vi "rsidr_core_global.vi"() -> ()   [LabVIEW 2020, in "Rohde&Schwarz RTx Oscilloscopes.lvlib"] (continued)
"Access"=0, "Range Table"="", "Read Callback"="rsrtx_FormatLINFrameRepCapInt_ReadCallback.vi", "Write Callback"="", "Supported Models"="", "Instrument Options"="", "Flags"=0, "Help"="Returns the checksum value.\n\nAvailable Repeated Capabilities:\nSerialBus: SB1, SB2, SB3, SB4\r\n\nRemote-control command(s):\nBUS<b>:LIN:FRAMe<n>:CSValue?"}, {"Level"=3, "Class Only"=FALSE, "Identifier"="RSRTX_ATTR_PROTOCOL_LIN_FRAME_PARITY_ENABLED", "Descriptive Name"="Protocol LIN Frame Parity Enabled", "Data Type"=0, "Command"="BUS{SerialBus}:LIN:FRAM<Frame>:IDST?", "Access"=0, "Range Table"="rsrtx_rngLINParity", "Read Callback"="rsrtx_FormatLINFrameRepCapInt_ReadCallback.vi", "Write Callback"="", "Supported Models"="", "Instrument Options"="", "Flags"=0, "Help"="Returns the identifier state of the selected frame.\n\nAvailable Repeated Capabilities:\nSerialBus: SB1, SB2, SB3, SB4\r\n\nRemote-control command(s):\nBUS<b>:LIN:FRAMe<n>:IDSTate?"}, {"Level"=3, "Class Only"=FALSE, "Identifier"="RSRTX_ATTR_PROTOCOL_LIN_FRAME_PARITY_VALUE", "Descriptive Name"="Protocol LIN Frame Parity Value", "Data Type"=0, "Command"="BUS{SerialBus}:LIN:FRAM<Frame>:IDPV?", "Access"=0, "Range Table"="", "Read Callback"="rsrtx_FormatLINFrameRepCapInt_ReadCallback.vi", "Write Callback"="", "Supported Models"="", "Instrument Options"="", "Flags"=0, "Help"="Returns the parity value.\n\nAvailable Repeated Capabilities:\nSerialBus: SB1, SB2, SB3, SB4\r\n\nRemote-control command(s):\nBUS<b>:LIN:FRAMe<n>:IDPValue?"}, {"Level"=3, "Class Only"=FALSE, "Identifier"="RSRTX_ATTR_PROTOCOL_LIN_FRAME_ID_VALUE", "Descriptive Name"="Protocol LIN Frame ID Value", "Data Type"=0, "Command"="BUS{SerialBus}:LIN:FRAM<Frame>:IDV?", "Access"=0, "Range Table"="", "Read Callback"="rsrtx_FormatLINFrameRepCapInt_ReadCallback.vi", "Write Callback"="", "Supported Models"="", "Instrument Options"="", "Flags"=0, "Help"="Returns the identifier value (address).\n\nAvailable Repeated Capabilities:\nSerialBus: SB1, SB2, SB3, SB4\r\n\nRemote-control command(s):\nBUS<b>:LIN:FRAMe<n>:IDValue?"}, {"Level"=3, "Class Only"=FALSE, "Identifier"="RSRTX_ATTR_PROTOCOL_LIN_FRAME_SYNC_ENABLED", "Descriptive Name"="Protocol LIN Frame Sync Enabled", "Data Type"=0, "Command"="BUS{SerialBus}:LIN:FRAM<Frame>:SYST?", "Access"=0, "Range Table"="rsrtx_rngLINChecksum", "Read Callback"="rsrtx_FormatLINFrameRepCapInt_ReadCallback.vi", "Write Callback"="", "Supported Models"="", "Instrument Options"="", "Flags"=0, "Help"="Returns the state of the sync field for the specified frame.\n\nAvailable Repeated Capabilities:\nSerialBus: SB1, SB2, SB3, SB4\r\n\nRemote-control command(s):\nBUS<b>:LIN:FRAMe<n>:SYSTate?"}, {"Level"=3, "Class Only"=FALSE, "Identifier"="RSRTX_ATTR_PROTOCOL_LIN_FRAME_SYNC_VALUE", "Descriptive Name"="Protocol LIN Frame Sync Value", "Data Type"=0, "Command"="BUS{SerialBus}:LIN:FRAM<Frame>:SYV?", "Access"=0, "Range Table"="", "Read Callback"="rsrtx_FormatLINFrameRepCapInt_ReadCallback.vi", "Write Callback"="", "Supported Models"="", "Instrument Options"="", "Flags"=0, "Help"="Returns the value of the synchronization field.\n\nAvailable Repeated Capabilities:\nSerialBus: SB1, SB2, SB3, SB4\r\n\nRemote-control command(s):\nBUS<b>:LIN:FRAMe<n>:SYValue?"}, {"Level"=3, "Class Only"=FALSE, "Identifier"="RSRTX_ATTR_PROTOCOL_LIN_FRAME_VERSION", "Descriptive Name"="Protocol LIN Frame Version", "Data Type"=0, "Command"="BUS{SerialBus}:LIN:FRAM<Frame>:VERS?", "Access"=0, "Range Table"="rsrtx_rngLINFrameVersion", "Read Callback"="rsrtx_FormatLINFrameRepCapInt_ReadCallback.vi", "Write Callback"="", "Supported Models"="", "Instrument Options"="", "Flags"=0, "Help"="Returns the version of the LIN standard for the specified frame.\n\nAvailable Repeated Capabilities:\nSerialBus: SB1, SB2, SB3, SB4\r\n\nRemote-control command(s):\nBUS<b>:LIN:FRAMe<n>:VERSion?"}, {"Level"=3, "Class Only"=FALSE, "Identifier"="RSRTX_ATTR_PROTOCOL_LIN_BYTE_COUNT", "Descriptive Name"="Protocol LIN Byte Count", "Data Type"=0, "Command"="BUS{SerialBus}:LIN:FRAM<Frame>:BCO?", "Access"=0, "Range Table"="", "Read Callback"="rsrtx_FormatLINFrameRepCapInt_ReadCallback.vi", "Write Callback"="", "Supported Models"="", "Instrument Options"="", "Flags"=0, "Help"="Returns the number of data bytes in the specified frame.\n\nAvailable Repeated Capabilities:\nSerialBus: SB1, SB2, SB3, SB4\r\n\nRemote-control command(s):\nBUS<b>:LIN:FRAMe<n>:BCOunt?"}, {"Level"=3, "Class Only"=FALSE, "Identifier"="RSRTX_ATTR_PROTOCOL_LIN_SELECTED_BYTE", "Descriptive Name"="Protocol LIN Selected Byte", "Data Type"=0, "Command"="", "Access"=2, "Range Table"="", "Read Callback"="", "Write Callback"="", "Supported Models"="", "Instrument Options"="", "Flags"=0, "Help"="Sets selector repeated capability Byte.\n\nAvailable Repeated Capabilities:\nNone\n\nRemote-control command(s):\n"}, {"Level"=3, "Class Only"=FALSE, "Identifier"="RSRTX_ATTR_PROTOCOL_LIN_BYTE_ENABLED", "Descriptive Name"="Protocol LIN Byte Enabled", "Data Type"=0, "Command"="BUS{SerialBus}:LIN:FRAM<Frame>:BYTE<Byte>:STAT?", "Access"=0, "Range Table"="rsrtx_rngLINByteEnabled", "Read Callback"="rsrtx_FormatLINFrameByteRepCapInt_ReadCallback.vi", "Write Callback"="", "Supported Models"="", "Instrument Options"="", "Flags"=0, "Help"="Returns the state of the specified data byte.\n\nAvailable Repeated Capabilities:\nSerialBus: SB1, SB2, SB3, SB4\r\n\nRemote-control command(s):\nBUS<b>:LIN:FRAMe<n>:BYTE<o>:STATe?"}, {"Level"=3, "Class Only"=FALSE, "Identifier"="RSRTX_ATTR_PROTOCOL_LIN_BYTE_VALUE", "Descriptive Name"="Protocol LIN Byte Value", "Data Type"=0, "Command"="BUS{SerialBus}:LIN:FRAM<Frame>:BYTE<Byte>:VAL?", "Access"=0, "Range Table"="", "Read Callback"="rsrtx_FormatLINFrameByteRepCapInt_ReadCallback.vi", "Write Callback"="", "Supported Models"="", "Instrument Options"="", "Flags"=0, "Help"="Returns the decimal value of the specified byte.\n\nAvailable Repeated Capabilities:\nSerialBus: SB1, SB2, SB3, SB4\r\n\nRemote-control command(s):\nBUS<b>:LIN:FRAMe<n>:BYTE<o>:VALue?"}, {"Level"=2, "Class Only"=TRUE, "Identifier"="", "Descriptive Name"="CAN", "Data Type"=0, "Command"="", "Access"=0, "Range Table"="", "Read Callback"="", "Write Callback"="", "Supported Models"="", "Instrument Options"="", "Flags"=0, "Help"="This class contains attributes that configure the CAN (Controller Area Network)\n\nAttributes in this class requires option K3."}, {"Level"=3, "Class Only"=FALSE, "Identifier"="RSRTX_ATTR_PROTOCOL_CAN_LINE_TYPE", "Descriptive Name"="Protocol CAN Line Type", "Data Type"=0, "Command"="BUS{SerialBus}:CAN:TYPE", "Access"=2, "Range Table"="rsrtx_rngProtocolCANLineType", "Read Callback"="", "Write Callback"="", "Supported Models"="", "Instrument Options"="K3", "Flags"=0, "Help"="Configures input channel of the CAN line.\n\nAvailable Repeated Capabilities:\nSerialBus: SB1, SB2, SB3, SB4\r\n\nRemote-control command(s):\nBUS<b>:CAN:TYPE"}, {"Level"=3, "Class Only"=FALSE, "Identifier"="RSRTX_ATTR_PROTOCOL_CAN_SOURCE", "Descriptive Name"="Protocol CAN Source", "Data Type"=0, "Command"="BUS{SerialBus}:CAN:DATA:SOUR", "Access"=2, "Range Table"="RsRtx_rngChannelAndDigitalSource", "Read Callback"="", "Write Callback"="", "Supported Models"="", "Instrument Options"="K3", "Flags"=0, "Help"="Configures source waveform of the data line.\n\nAvailable Repeated Capabilities:\nSerialBus: SB1, SB2, SB3, SB4\r\n\nRemote-control command(s):\nBUS<b>:CAN:DATA:SOURce"}, {"Level"=3, "Class Only"=FALSE, "Identifier"="RSRTX_ATTR_PROTOCOL_CAN_BIT_RATE", "Descriptive Name"="Protocol CAN Bit Rate", "Data Type"=1, "Command"="BUS{SerialBus}:CAN:BITR", "Access"=2, "Range Table"="rsrtx_rngProtocolCANBitRate", "Read Callback"="", "Write Callback"="", "Supported Models"="", "Instrument Options"="K3", "Flags"=0, "Help"="Sets the number of transmitted bits per second.\n\nAvailable Repeated Capabilities:\nSerialBus: SB1, SB2, SB3, SB4\r\n\nRemote-control command(s):\nBUS<b>:CAN:BITRate"}, {"Level"=3, "Class Only"=FALSE, "Identifier"="RSRTX_ATTR_PROTOCOL_CAN_SAMPLE_POINT", "Descriptive Name"="Protocol CAN Sample Point", "Data Type"=1, "Command"="BUS{SerialBus}:CAN:SAMP", "Access"=2, "Range Table"="rsrtx_rngProtocolCANSamplePoint", "Read Callback"="", "Write Callback"="", "Supported Models"="", "Instrument Options"="K3", "Flags"=0, "Help"="Sets the position of the sample point within the bit in percent of the nominal bit time.\n\nAvailable Repeated Capabilities:\nSerialBus: SB1, SB2, SB3, SB4\r\n\nRemote-control command(s):\nBUS<b>:CAN:SAMPlepoint"}, {"Level"=3, "Class Only"=FALSE, "Identifier"="RSRTX_ATTR_PROTOCOL_CAN_FRAME_COUNT", "Descriptive Name"="Protocol CAN Frame Count", "Data Type"=0, "Command"="BUS{SerialBus}:CAN:FCO?", "Access"=0, "Range Table"="", "Read Callback"="", "Write Callback"="", "Supported Models"="", "Instrument Options"="K3", "Flags"=0, "Help"="Queries the number of decoded frames.\n\nAvailable Repeated Capabilities:\nSerialBus: SB1, SB2, SB3, SB4\r\n\nRemote-control command(s):\nBUS<b>:CAN:FCOunt?"}, {"Level"=3, "Class Only"=FALSE, "Identifier"="RSRTX_ATTR_PROTOCOL_CAN_SELECTED_FRAME", "Descriptive Name"="Protocol CAN Selected Frame", "Data Type"=0, "Command"="", "Access"=2, "Range Table"="", "Read Callback"="", "Write Callback"="", "Supported Models"="", "Instrument Options"="", "Flags"=0, "Help"="Sets selector repeated capability Frame.\n\nAvailable Repeated Capabilities:\nNone\n\nRemote-control command(s):\n"}, {"Level"=3, "Class Only"=FALSE, "Identifier"="RSRTX_ATTR_PROTOCOL_CAN_FRAME_TYPE", "Descriptive Name"="Protocol CAN Frame Type", "Data Type"=0, "Command"="BUS{SerialBus}:CAN:FRAM<Frame>:TYPE?", "Access"=0, "Range Table"="rsrtx_rngCANFrameType", "Read Callback"="rsrtx_FormatCANFrameRepCapInt_ReadCallback.vi", "Write Callback"="", "Supported Models"="", "Instrument Options"="", "Flags"=0, "Help"="Returns the type of the specified frame.\n\nAvailable Repeated Capabilities:\nSerialBus: SB1, SB2, SB3, SB4\r\n\nRemote-control command(s):\nBUS<b>:CAN:FRAMe<n>:TYPE?"}, {"Level"=3, "Class Only"=FALSE, "Identifier"="RSRTX_ATTR_PROTOCOL_CAN_FRAME_STATUS", "Descriptive Name"="Protocol CAN Frame Status", "Data Type"=0, "Command"="BUS{SerialBus}:CAN:FRAM<Frame>:STATus?", "Access"=0, "Range Table"="rsrtx_rngCANFrameStatus", "Read Callback"="rsrtx_FormatCANFrameRepCapInt_ReadCallback.vi", "Write Callback"="", "Supported Models"="", "Instrument Options"="", "Flags"=0, "Help"="Returns the overall state of the specified frame.\n\nAvailable Repeated Capabilities:\nSerialBus: SB1, SB2, SB3, SB4\r\n\nRemote-control command(s):\nBUS<b>:CAN:FRAMe<n>:STATus?"}, {"Level"=3, "Class Only"=FALSE, "Identifier"="RSRTX_ATTR_PROTOCOL_CAN_FRAME_START", "Descriptive Name"="Protocol CAN Frame Start", "Data Type"=1, "Command"="BUS{SerialBus}:CAN:FRAM<Frame>:STAR?", "Access"=0, "Range Table"="", "Read Callback"="rsrtx_FormatCANFrameRepCapReal_ReadCallback.vi", "Write Callback"="", "Supported Models"="", "Instrument Options"="", "Flags"=0, "Help"="Returns the start time of the specified frame.\n\nAvailable Repeated Capabilities:\nSerialBus: SB1, SB2, SB3, SB4\r\n\nRemote-control command(s):\nBUS<b>:CAN:FRAMe<n>:STARt?"}, {"Level"=3, "Class Only"=FALSE, "Identifier"="RSRTX_ATTR_PROTOCOL_CAN_FRAME_END", "Descriptive Name"="Protocol CAN Frame End", "Data Type"=1, "Command"="BUS{SerialBus}:CAN:FRAM<Frame>:STOP?", "Access"=0, "Range Table"="", "Read Callback"="rsrtx_FormatCANFrameRepCapReal_ReadCallback.vi", "Write Callback"="", "Supported Models"="", "Instrument Options"="", "Flags"=0, "Help"="Returns the end time of the specified frame.\n\nAvailable Repeated Capabilities:\nSerialBus: SB1, SB2, SB3, SB4\r\n\nRemote-control command(s):\nBUS<b>:CAN:FRAMe<n>:STOP?"}, {"Level"=3, "Class Only"=FALSE, "Identifier"="RSRTX_ATTR_PROTOCOL_CAN_FRAME_DATA", "Descriptive Name"="Protocol CAN Frame Data", "Data Type"=2, "Command"="BUS{SerialBus}:CAN:FRAM<Frame>:DATA?", "Access"=0, "Range Table"="", "Read Callback"="rsrtx_FormatCANFrameRepCapString_ReadCallback.vi", "Write Callback"="", "Supported Models"="", "Instrument Options"="", "Flags"=0, "Help"="Returns the data words of the specified frame.\n\nAvailable Repeated Capabilities:\nSerialBus: SB1, SB2, SB3, SB4\r\n\nRemote-control command(s):\nBUS<b>:CAN:FRAMe<n>:DATA?"}, {"Level"=3, "Class Only"=FALSE, "Identifier"="RSRTX_ATTR_PROTOCOL_CAN_ACK_STATE", "Descriptive Name"="Protocol CAN Ack State", "Data Type"=0, "Command"="BUS{SerialBus}:CAN:FRAM<Frame>:ACKS?", "Access"=0, "Range Table"="rsrtx_rngCANAckState", "Read Callback"="rsrtx_FormatCANFrameRepCapInt_ReadCallback.vi", "Write Callback"="", "Supported Models"="", "Instrument Options"="", "Flags"=0, "Help"="Returns the state of the acknowledge field.\n\nAvailable Repeated Capabilities:\nSerialBus: SB1, SB2, SB3, SB4\r\n\nRemote-control command(s):\nBUS<b>:CAN:FRAMe<n>:ACKState?"}, {"Level"=3, "Class Only"=FALSE, "Identifier"="RSRTX_ATTR_PROTOCOL_CAN_ACK_VALUE", "Descriptive Name"="Protocol CAN Ack Value", "Data Type"=0, "Command"="BUS{SerialBus}:CAN:FRAM<Frame>:ACKV?", "Access"=0, "Range Table"="", "Read Callback"="rsrtx_FormatCANFrameRepCapInt_ReadCallback.vi", "Write Callback"="", "Supported Models"="", "Instrument Options"="", "Flags"=0, "Help"="Returns the value of the acknowledge field.\n\nAvailable Repeated Capabilities:\nSerialBus: SB1, SB2, SB3, SB4\r\n\nRemote-control command(s):\nBUS<b>:CAN:FRAMe<n>:ACKValue?"}, {"Level"=3, "Class Only"=FALSE, "Identifier"="RSRTX_ATTR_PROTOCOL_CAN_CHECKSUM_STATE", "Descriptive Name"="Protocol CAN Checksum State", "Data Type"=0, "Command"="BUS{SerialBus}:CAN:FRAM<Frame>:CSST?", "Access"=0, "Range Table"="rsrtx_rngCANAckState", "Read Callback"="rsrtx_FormatCANFrameRepCapInt_ReadCallback.vi", "Write Callback"="", "Supported Models"="", "Instrument Options"="", "Flags"=0, "Help"="Returns the state of the checksum.\n\nAvailable Repeated Capabilities:\nSerialBus: SB1, SB2, SB3, SB4\r\n\nRemote-control command(s):\nBUS<b>:CAN:FRAMe<n>:CSSTate?"}, {"Level"=3, "Class Only"=FALSE, "Identifier"="RSRTX_ATTR_PROTOCOL_CAN_CHECKSUM_VALUE", "Descriptive Name"="Protocol CAN Checksum Value", "Data Type"=0, "Command"="BUS{SerialBus}:CAN:FRAM<Frame>:CSV?", "Access"=0, "Range Table"="", "Read Callback"="rsrtx_FormatCANFrameRepCapInt_ReadCallback.vi", "Write Callback"="", "Supported Models"="", "Instrument Options"="", "Flags"=0, "Help"="Returns the checksum value.\n\nAvailable Repeated Capabilities:\nSerialBus: SB1, SB2, SB3, SB4\r\n\nRemote-control command(s):\nBUS<b>:CAN:FRAMe<n>:CSValue?"}, {"Level"=3, "Class Only"=FALSE, "Identifier"="RSRTX_ATTR_PROTOCOL_CAN_DATA_LENGTH_STATE", "Descriptive Name"="Protocol CAN Data Length State", "Data Type"=0, "Command"="BUS{SerialBus}:CAN:FRAM<Frame>:DLCS?", "Access"=0, "Range Table"="rsrtx_rngCANAckState", "Read Callback"="rsrtx_FormatCANFrameRepCapInt_ReadCallback.vi", "Write Callback"="", "Supported Models"="", "Instrument Options"="", "Flags"=0, "Help"="Returns the state of the data length code.\n\nAvailable Repeated Capabilities:\nSerialBus: SB1, SB2, SB3, SB4\r\n\nRemote-control command(s):\nBUS<b>:CAN:FRAMe<n>:DLCState?"}, {"Level"=3, "Class Only"=FALSE, "Identifier"="RSRTX_ATTR_PROTOCOL_CAN_DATA_LENGTH_VALUE", "Descriptive Name"="Protocol CAN Data Length Value", "Data Type"=0, "Command"="BUS{SerialBus}:CAN:FRAM<Frame>:DLCV?", "Access"=0, "Range Table"="", "Read Callback"="rsrtx_FormatCANFrameRepCapInt_ReadCallback.vi", "Write Callback"="", "Supported Models"="", "Instrument Options"="", "Flags"=0, "Help"="Returns the number of data bytes in the specified frame.\n\nAvailable Repeated Capabilities:\nSerialBus: SB1, SB2, SB3, SB4\r\n\nRemote-control command(s):\nBUS<b>:CAN:FRAMe<n>:DLCValue?"}, {"Level"=3, "Class Only"=FALSE, "Identifier"="RSRTX_ATTR_PROTOCOL_CAN_ID_STATE", "Descriptive Name"="Protocol CAN ID State", "Data Type"=0, "Command"="BUS{SerialBus}:CAN:FRAM<Frame>:IDST?", "Access"=0, "Range Table"="rsrtx_rngCANAckState", "Read Callback"="rsrtx_FormatCANFrameRepCapInt_ReadCallback.vi", "Write Callback"="", "Supported Models"="", "Instrument Options"="", "Flags"=0, "Help"="Returns the state of the identifier.\n\nAvailable Repeated Capabilities:\nSerialBus: SB1, SB2, SB3, SB4\r\n\nRemote-control command(s):\nBUS<b>:CAN:FRAMe<n>:IDSTate?"}, {"Level"=3, "Class Only"=FALSE, "Identifier"="RSRTX_ATTR_PROTOCOL_CAN_ID_VALUE", "Descriptive Name"="Protocol CAN ID Value", "Data Type"=0, "Command"="BUS{SerialBus}:CAN:FRAM<Frame>:IDV?", "Access"=0, "Range Table"="", "Read Callback"="rsrtx_FormatCANFrameRepCapInt_ReadCallback.vi", "Write Callback"="", "Supported Models"="", "Instrument Options"="", "Flags"=0, "Help"="Returns the decimal address value of the specified frame.\n\nAvailable Repeated Capabilities:\nSerialBus: SB1, SB2, SB3, SB4\r\n\nRemote-control command(s):\nBUS<b>:CAN:FRAMe<n>:IDValue?"}, {"Level"=3, "Class Only"=FALSE, "Identifier"="RSRTX_ATTR_PROTOCOL_CAN_ID_TYPE", "Descriptive Name"="Protocol CAN ID Type", "Data Type"=0, "Command"="BUS{SerialBus}:CAN:FRAM<Frame>:IDTY?", "Access"=0, "Range Table"="rsrtx_rngProtocolCANIDType", "Read Callback"="rsrtx_FormatCANFrameRepCapInt_ReadCallback.vi", "Write Callback"="", "Supported Models"="", "Instrument Options"="", "Flags"=0, "Help"="Returns the length of the identifier: 11 bit for CAN base frames, or 29 bits for CAN extended frames.\n\nAvailable Repeated Capabilities:\nSerialBus: SB1, SB2, SB3, SB4\r\n\nRemote-control command(s):\nBUS<b>:CAN:FRAMe<n>:IDTYpe?"}, {"Level"=3, "Class Only"=FALSE, "Identifier"="RSRTX_ATTR_PROTOCOL_CAN_BSE_POSITION", "Descriptive Name"="Protocol CAN BSE Position", "Data Type"=1, "Command"="BUS{SerialBus}:CAN:FRAM<Frame>:BSEP?", "Access"=0, "Range Table"="", "Read Callback"="rsrtx_FormatCANFrameRepCapReal_ReadCallback.vi", "Write Callback"="", "Supported Models"="", "Instrument Options"="", "Flags"=0, "Help"="Returns the position of the bit stuffing error in the specified frame (if available).\n\nAvailable Repeated Capabilities:\nSerialBus: SB1, SB2, SB3, SB4\r\n\nRemote-control command(s):\nBUS<b>:CAN:FRAMe<n>:BSEPosition?"}, {"Level"=3, "Class Only"=FALSE, "Identifier"="RSRTX_ATTR_PROTOCOL_CAN_BYTE_COUNT", "Descriptive Name"="Protocol CAN Byte Count", "Data Type"=0, "Command"="BUS{SerialBus}:CAN:FRAM<Frame>:BCO?", "Access"=0, "Range Table"="", "Read Callback"="rsrtx_FormatCANFrameRepCapInt_ReadCallback.vi", "Write Callback"="", "Supported Models"="", "Instrument Options"="", "Flags"=0, "Help"="Returns the number of data bytes in the specified frame.\n\nAvailable Repeated Capabilities:\nSerialBus: SB1, SB2, SB3, SB4\r\n\nRemote-control command(s):\nBUS<b>:CAN:FRAMe<n>:BCOunt?"}, {"Level"=3, "Class Only"=FALSE, "Identifier"="RSRTX_ATTR_PROTOCOL_CAN_SELECTED_BYTE", "Descriptive Name"="Protocol CAN Selected Byte", "Data Type"=0, "Command"="", "Access"=2, "Range Table"="", "Read Callback"="", "Write Callback"="", "Supported Models"="", "Instrument Options"="", "Flags"=0, "Help"="Sets selector repeated capability Byte.\n\nAvailable Repeated Capabilities:\nNone\n\nRemote-control command(s):\n"}, {"Level"=3, "Class Only"=FALSE, "Identifier"="RSRTX_ATTR_PROTOCOL_CAN_BYTE_STATE", "Descriptive Name"="Protocol CAN Byte State", "Data Type"=0, "Command"="BUS{SerialBus}:CAN:FRAM<Frame>:BYTE<Byte>:STAT?", "Access"=0, "Range Table"="rsrtx_rngCANAckState", "Read Callback"="rsrtx_FormatCANFrameByteRepCapInt_ReadCallback.vi", "Write Callback"="", "Supported Models"="", "Instrument Options"="", "Flags"=0, "Help"="Returns the state of the specified data byte.\n\nAvailable Repeated Capabilities:\nSerialBus: SB1, SB2, SB3, SB4\r\n\nRemote-control command(s):\nBUS<b>:CAN:FRAMe<n>:BYTE<o>:STATe?"}, {"Level"=3, "Class Only"=FALSE, "Identifier"="RSRTX_ATTR_PROTOCOL_CAN_BYTE_VALUE", "Descriptive Name"="Protocol CAN Byte Value", "Data Type"=0, "Command"="BUS{SerialBus}:CAN:FRAM<Frame>:BYTE<Byte>:VALue?", "Access"=0, "Range Table"="", "Read Callback"="rsrtx_FormatCANFrameByteRepCapInt_ReadCallback.vi", "Write Callback"="", "Supported Models"="", "Instrument Options"="", "Flags"=0, "Help"="Returns the decimal value of the specified byte.\n\nAvailable Repeated Capabilities:\nSerialBus: SB1, SB2, SB3, SB4\r\n\nRemote-control command(s):\nBUS<b>:CAN:FRAMe<n>:BYTE<o>:VALue?"}, {"Level"=2, "Class Only"=TRUE, "Identifier"="", "Descriptive Name"="Parallel Bus", "Data Type"=0, "Command"="", "Access"=0, "Range Table"="", "Read Callback"="", "Write Callback"="", "Supported Models"="", "Instrument Options"="", "Flags"=0, "Help"="Parallel Bus settings."}, {"Level"=3, "Class Only"=FALSE, "Identifier"="RSRTX_ATTR_PARALLEL_BUS_ANALYZED_LINES", "Descriptive Name"="Parallel Bus Analyzed Lines", "Data Type"=0, "Command"="BUS{SerialBus}:PAR:WIDT", "Access"=2, "Range Table"="rsrtx_rngParallelBusAnalyzedLines", "Read Callback"="", "Write Callback"="", "Supported Models"="", "Instrument Options"="", "Flags"=0, "Help"="Sets the number of lines to be analyzed.\n\nAvailable Repeated Capabilities:\nSerialBus: SB1, SB2, SB3, SB4\r\n\nRemote-control command(s):\nBUS<b>:PARallel:WIDTh"}, {"Level"=3, "Class Only"=FALSE, "Identifier"="RSRTX_ATTR_PARALLEL_BUS_FRAME_COUNT", "Descriptive Name"="Parallel Bus Frame Count", "Data Type"=0, "Command"="BUS{SerialBus}:PAR:FCO?", "Access"=0, "Range Table"="", "Read Callback"="", "Write Callback"="", "Supported Models"="", "Instrument Options"="", "Flags"=0, "Help"="Returns the number of decoded frames.\n\nAvailable Repeated Capabilities:\nSerialBus: SB1, SB2, SB3, SB4\r\n\nRemote-control command(s):\nBUS<b>:PARallel:FCOunt?"}, {"Level"=3, "Class Only"=FALSE, "Identifier"="RSRTX_ATTR_PARALLEL_BUS_SELECTED_FRAME", "Descriptive Name"="Parallel Bus Selected Frame", "Data Type"=0, "Command"="", "Access"=2, "Range Table"="", "Read Callback"="", "Write Callback"="", "Supported Models"="", "Instrument Options"="", "Flags"=0, "Help"="Sets selector repeated capability Frame.\n\nAvailable Repeated Capabilities:\nNone\n\nRemote-control command(s):\n"}, {"Level"=3, "Class Only"=FALSE, "Identifier"="RSRTX_ATTR_PARALLEL_BUS_FRAME_DATA", "Descriptive Name"="Parallel Bus Frame Data", "Data Type"=2, "Command"="BUS{SerialBus}:PAR:FRAM<Frame>:DATA?", "Access"=0, "Range Table"="", "Read Callback"="rsrtx_FormatParallelFrameRepCapString_ReadCallback.vi", "Write Callback"="", "Supported Models"="", "Instrument Options"="", "Flags"=0, "Help"="Returns the data words of the specified frame.\n\nAvailable Repeated Capabilities:\nSerialBus: SB1, SB2, SB3, SB4\r\n\nRemote-control command(s):\nBUS<b>:PARallel:FRAMe<n>:DATA?"}, {"Level"=3, "Class Only"=FALSE, "Identifier"="RSRTX_ATTR_PARALLEL_BUS_FRAME_ENABLED", "Descriptive Name"="Parallel Bus Frame Enabled", "Data Type"=0, "Command"="BUS{SerialBus}:PAR:FRAM<Frame>:STAT?", "Access"=0, "Range Table"="rsrtx_rngParallelBusFrameEnabled", "Read Callback"="rsrtx_FormatParallelFrameRepCapInt_ReadCallback.vi", "Write Callback"="", "Supported Models"="", "Instrument Options"="", "Flags"=0, "Help"="Returns the overall state of the specified frame.\n\nAvailable Repeated Capabilities:\nSerialBus: SB1, SB2, SB3, SB4\r\n\nRemote-control command(s):\nBUS<b>:PARallel:FRAMe<n>:STATe?"}, {"Level"=3, "Class Only"=FALSE, "Identifier"="RSRTX_ATTR_PARALLEL_BUS_FRAME_START", "Descriptive Name"="Parallel Bus Frame Start", "Data Type"=1, "Command"="BUS{SerialBus}:PAR:FRAM<Frame>:STAR?", "Access"=0, "Range Table"="", "Read Callback"="rsrtx_FormatParallelFrameRepCapReal_ReadCallback.vi", "Write Callback"="", "Supported Models"="", "Instrument Options"="", "Flags"=0, "Help"="Returns the start time of the specified frame.\n\nAvailable Repeated Capabilities:\nSerialBus: SB1, SB2, SB3, SB4\r\n\nRemote-control command(s):\nBUS<b>:PARallel:FRAMe<n>:STARt?"}, {"Level"=3, "Class Only"=FALSE, "Identifier"="RSRTX_ATTR_PARALLEL_BUS_FRAME_END", "Descriptive Name"="Parallel Bus Frame End", "Data Type"=1, "Command"="BUS{SerialBus}:PAR:FRAM<Frame>:STOP?", "Access"=0, "Range Table"="", "Read Callback"="rsrtx_FormatParallelFrameRepCapReal_ReadCallback.vi", "Write Callback"="", "Supported Models"="", "Instrument Options"="", "Flags"=0, "Help"="Returns the end time of the specified frame.\n\nAvailable Repeated Capabilities:\nSerialBus: SB1, SB2, SB3, SB4\r\n\nRemote-control command(s):\nBUS<b>:PARallel:FRAMe<n>:STOP?"}, {"Level"=3, "Class Only"=TRUE, "Identifier"="", "Descriptive Name"="Line", "Data Type"=0, "Command"="", "Access"=0, "Range Table"="", "Read Callback"="", "Write Callback"="", "Supported Models"="", "Instrument Options"="", "Flags"=0, "Help"="This class contains methods for configuring individual lines of the parallel bus."}, {"Level"=4, "Class Only"=FALSE, "Identifier"="RSRTX_ATTR_PARALLEL_BUS_BIT_SOURCE", "Descriptive Name"="Parallel Bus Bit Source", "Data Type"=0, "Command"="BUS{SerialBus}:PAR:DATA{ParallelLine}:SOUR", "Access"=2, "Range Table"="RsRtx_rngParallelBitSource", "Read Callback"="", "Write Callback"="", "Supported Models"="", "Instrument Options"="", "Flags"=0, "Help"="Defines the logic channel that is assigned to the selected bit. Use the command for each bit of the bus.\n\nAvailable Repeated Capabilities:\nSerialBus: SB1, SB2, SB3, SB4\r\nParallelLine: Bit0, Bit1, Bit2, Bit3, Bit4, Bit5, Bit6, Bit7, Bit8, Bit9, Bit10, Bit11, Bit12, Bit13, Bit14, Bit15\r\n\nRemote-control command(s):\nBUS<b>:PARallel:DATA<m>:SOURce"}, {"Level"=3, "Class Only"=TRUE, "Identifier"="", "Descriptive Name"="Parallel Bus Clocked", "Data Type"=0, "Command"="", "Access"=0, "Range Table"="", "Read Callback"="", "Write Callback"="", "Supported Models"="", "Instrument Options"="", "Flags"=0, "Help"="Parallel Bus clocked settings."}, {"Level"=4, "Class Only"=FALSE, "Identifier"="RSRTX_ATTR_PARALLEL_BUS_CLOCKED_ANALYZED_LINES", "Descriptive Name"="Parallel Bus Clocked Analyzed Lines", "Data Type"=0, "Command"="BUS{SerialBus}:CPAR:WIDT", "Access"=2, "Range Table"="rsrtx_rngParallelBusAnalyzedLines", "Read Callback"="", "Write Callback"="", "Supported Models"="", "Instrument Options"="", "Flags"=0, "Help"="Sets the number of lines to be analyzed.\n\nAvailable Repeated Capabilities:\nSerialBus: SB1, SB2, SB3, SB4\r\n\nRemote-control command(s):\nBUS<b>:CPARallel:WIDTh"}, {"Level"=4, "Class Only"=FALSE, "Identifier"="RSRTX_ATTR_PARALLEL_BUS_CLOCKED_FRAME_COUNT", "Descriptive Name"="Parallel Bus Clocked Frame Count", "Data Type"=0, "Command"="BUS{SerialBus}:CPAR:FCO?", "Access"=0, "Range Table"="", "Read Callback"="", "Write Callback"="", "Supported Models"="", "Instrument Options"="", "Flags"=0, "Help"="Returns the number of decoded frames.\n\nAvailable Repeated Capabilities:\nSerialBus: SB1, SB2, SB3, SB4\r\n\nRemote-control command(s):\nBUS<b>:CPARallel:FCOunt?"}, {"Level"=4, "Class Only"=FALSE, "Identifier"="RSRTX_ATTR_PARALLEL_BUS_CLOCKED_SLOPE", "Descriptive Name"="Parallel Bus Clocked Slope", "Data Type"=0, "Command"="BUS{SerialBus}:CPAR:CLOCK:SLOP", "Access"=2, "Range Table"="rsrtx_rngTriggerSlope", "Read Callback"="", "Write Callback"="", "Supported Models"="", "Instrument Options"="", "Flags"=0, "Help"="Selects if the data is sampled on the rising or falling slope of the clock, or on both edges (EITHer). The clock slope marks the begin of a new bit.\n\nAvailable Repeated Capabilities:\nSerialBus: SB1, SB2, SB3, SB4\r\n\nRemote-control command(s):\nBUS<b>:CPARallel:CLOCK:SLOPe"}, {"Level"=4, "Class Only"=FALSE, "Identifier"="RSRTX_ATTR_PARALLEL_BUS_CLOCKED_CS_POLARITY", "Descriptive Name"="Parallel Bus Clocked CS Polarity", "Data Type"=0, "Command"="BUS{SerialBus}:CPAR:CS:POL", "Access"=2, "Range Table"="rsrtx_rngPolarity", "Read Callback"="", "Write Callback"="", "Supported Models"="", "Instrument Options"="", "Flags"=0, "Help"="Selects wether the chip select signal is high active (high = 1) or low active (low = 1).\n\nAvailable Repeated Capabilities:\nSerialBus: SB1, SB2, SB3, SB4\r\n\nRemote-control command(s):\nBUS<b>:CPARallel:CS:POLarity"}, {"Level"=4, "Class Only"=FALSE, "Identifier"="RSRTX_ATTR_PARALLEL_BUS_CLOCKED_SELECTED_FRAME", "Descriptive Name"="Parallel Bus Clocked Selected Frame", "Data Type"=0, "Command"="", "Access"=2, "Range Table"="", "Read Callback"="", "Write Callback"="", "Supported Models"="", "Instrument Options"="", "Flags"=0, "Help"="Sets selector repeated capability Frame.\n\nAvailable Repeated Capabilities:\nNone\n\nRemote-control command(s):\n"}, {"Level"=4, "Class Only"=FALSE, "Identifier"="RSRTX_ATTR_PARALLEL_BUS_CLOCKED_FRAME_DATA", "Descriptive Name"="Parallel Bus Clocked Frame Data", "Data Type"=2, "Command"="BUS{SerialBus}:CPAR:FRAM<Frame>:DATA?", "Access"=0, "Range Table"="", "Read Callback"="rsrtx_FormatClockedFrameRepCapString_ReadCallback.vi", "Write Callback"="", "Supported Models"="", "Instrument Options"="", "Flags"=0, "Help"="Returns the data words of the specified frame.\n\nAvailable Repeated Capabilities:\nSerialBus: SB1, SB2, SB3, SB4\r\n\nRemote-control command(s):\nBUS<b>:CPARallel:FRAMe<n>:DATA?"}, {"Level"=4, "Class Only"=FALSE, "Identifier"="RSRTX_ATTR_PARALLEL_BUS_CLOCKED_FRAME_ENABLED", "Descriptive Name"="Parallel Bus Clocked Frame Enabled", "Data Type"=0, "Command"="BUS{SerialBus}:CPAR:FRAM<Frame>:STAT?", "Access"=0, "Range Table"="rsrtx_rngParallelBusFrameEnabled", "Read Callback"="rsrtx_FormatClockedFrameRepCapInt_ReadCallback.vi", "Write Callback"="", "Supported Models"="", "Instrument Options"="", "Flags"=0, "Help"="Returns the overall state of the specified frame.\n\nAvailable Repeated Capabilities:\nSerialBus: SB1, SB2, SB3, SB4\r\n\nRemote-control command(s):\nBUS<b>:CPARallel:FRAMe<n>:STATe?"}, {"Level"=4, "Class Only"=FALSE, "Identifier"="RSRTX_ATTR_PARALLEL_BUS_CLOCKED_FRAME_START", "Descriptive Name"="Parallel Bus Clocked Frame Start", "Data Type"=1, "Command"="BUS{SerialBus}:CPAR:FRAM<Frame>:STAR?", "Access"=0, "Range Table"="", "Read Callback"="rsrtx_FormatClockedFrameRepCapReal_ReadCallback.vi", "Write Callback"="", "Supported Models"="", "Instrument Options"="", "Flags"=0, "Help"="Returns the start time of the specified frame.\n\nAvailable Repeated Capabilities:\nSerialBus: SB1, SB2, SB3, SB4\r\n\nRemote-control command(s):\nBUS<b>:CPARallel:FRAMe<n>:STARt?"}, {"Level"=4, "Class Only"=FALSE, "Identifier"="RSRTX_ATTR_PARALLEL_BUS_CLOCKED_FRAME_END", "Descriptive Name"="Parallel Bus Clocked Frame End", "Data Type"=1, "Command"="BUS{SerialBus}:CPAR:FRAM<Frame>:STOP?", "Access"=0, "Range Table"="", "Read Callback"="rsrtx_FormatClockedFrameRepCapReal_ReadCallback.vi", "Write Callback"="", "Supported Models"="", "Instrument Options"="", "Flags"=0, "Help"="Returns the end time of the specified frame.\n\nAvailable Repeated Capabilities:\nSerialBus: SB1, SB2, SB3, SB4\r\n\nRemote-control command(s):\nBUS<b>:CPARallel:FRAMe<n>:STOP?"}, {"Level"=4, "Class Only"=FALSE, "Identifier"="RSRTX_ATTR_PARALLEL_BUS_CLOCKED_SOURCE", "Descriptive Name"="Parallel Bus Clocked Source", "Data Type"=0, "Command"="BUS{SerialBus}:CPAR:CLOC:SOUR", "Access"=2, "Range Table"="RsRtx_rngClockedSource", "Read Callback"="", "Write Callback"="", "Supported Models"="", "Instrument Options"="", "Flags"=0, "Help"="Selects the digital channel that is used as clock line.\n\nAvailable Repeated Capabilities:\nSerialBus: SB1, SB2, SB3, SB4\r\n\nRemote-control command(s):\nBUS<b>:CPARallel:CLOCk:SOURce"}, {"Level"=4, "Class Only"=FALSE, "Identifier"="RSRTX_ATTR_PARALLEL_BUS_CLOCKED_CHIP_SELECT_ENABLED", "Descriptive Name"="Parallel Bus Clocked Chip Select Enabled", "Data Type"=3, "Command"="BUS{SerialBus}:CPAR:CS:ENAB", "Access"=2, "Range Table"="", "Read Callback"="", "Write Callback"="", "Supported Models"="", "Instrument Options"="", "Flags"=0, "Help"="Enables and disables the chip select line.\n\nAvailable Repeated Capabilities:\nSerialBus: SB1, SB2, SB3, SB4\r\n\nRemote-control command(s):\nBUS<b>:CPARallel:CS:ENABle"}, {"Level"=4, "Class Only"=FALSE, "Identifier"="RSRTX_ATTR_PARALLEL_BUS_CLOCKED_CHIP_SELECT_SOURCE", "Descriptive Name"="Parallel Bus Clocked Chip Select Source", "Data Type"=0, "Command"="BUS{SerialBus}:CPAR:CS:SOUR", "Access"=2, "Range Table"="RsRtx_rngClockedSource", "Read Callback"="", "Write Callback"="", "Supported Models"="", "Instrument Options"="", "Flags"=0, "Help"="Selects the digital channel that is used as chip select line.\n\nAvailable Repeated Capabilities:\nSerialBus: SB1, SB2, SB3, SB4\r\n\nRemote-control command(s):\nBUS<b>:CPARallel:CS:SOURce"}, {"Level"=4, "Class Only"=TRUE, "Identifier"="", "Descriptive Name"="Line", "Data Type"=0, "Command"="", "Access"=0, "Range Table"="", "Read Callback"="", "Write Callback"="", "Supported Models"="", "Instrument Options"="", "Flags"=0, "Help"="This class contains methods for configuring individual lines of the parallel bus."}, {"Level"=5, "Class Only"=FALSE, "Identifier"="RSRTX_ATTR_PARALLEL_BUS_CLOCKED_BIT_SOURCE", "Descriptive Name"="Parallel Bus Clocked Bit Source", "Data Type"=0, "Command"="BUS{SerialBus}:CPAR:DATA{ParallelLine}:SOUR", "Access"=2, "Range Table"="RsRtx_rngParallelBitSource", "Read Callback"="", "Write Callback"="", "Supported Models"="", "Instrument Options"="", "Flags"=0, "Help"="Defines the logic channel that is assigned to the selected bit. Use the command for each bit of the bus.\n\nAvailable Repeated Capabilities:\nSerialBus: SB1, SB2, SB3, SB4\r\nParallelLine: Bit0, Bit1, Bit2, Bit3, Bit4, Bit5, Bit6, Bit7, Bit8, Bit9, Bit10, Bit11, Bit12, Bit13, Bit14, Bit15\r\n\nRemote-control command(s):\nBUS<b>:CPARallel:DATA<m>:SOURce"}, {"Level"=2, "Class Only"=TRUE, "Identifier"="", "Descriptive Name"="Audio Signals", "Data Type"=0, "Command"="", "Access"=0, "Range Table"="", "Read Callback"="", "Write Callback"="", "Supported Models"="", "Instrument Options"="", "Flags"=0, "Help"="This class contains attributes that configure and analyze audio signals. \n\nAttributes in this class requires option R&S RTO-K5."}, {"Level"=3, "Class Only"=FALSE, "Identifier"="RSRTX_ATTR_PROTOCOL_AUDIO_VARIANT", "Descriptive Name"="Protocol Audio Variant", "Data Type"=0, "Command"="BUS{SerialBus}:I2S:AVAR", "Access"=2, "Range Table"="rsrtx_rngAudioVariant", "Read Callback"="", "Write Callback"="", "Supported Models"="RTM|RTA", "Instrument Options"="", "Flags"=0, "Help"="Selects the audio signal type.\n\nAvailable Repeated Capabilities:\nSerialBus: SB1, SB2, SB3, SB4\r\n\nRemote-control command(s):\nBUS<b>:I2S:AVARiant"}, {"Level"=3, "Class Only"=FALSE, "Identifier"="RSRTX_ATTR_PROTOCOL_AUDIO_WORD_LENGTH", "Descriptive Name"="Protocol Audio Word Length", "Data Type"=0, "Command"="BUS{SerialBus}:I2S:WLEN", "Access"=2, "Range Table"="", "Read Callback"="", "Write Callback"="", "Supported Models"="RTM|RTA", "Instrument Options"="", "Flags"=0, "Help"="Defines the number of bits in an audio data word.\n\nAvailable Repeated Capabilities:\nSerialBus: SB1, SB2, SB3, SB4\r\n\nRemote-control command(s):\nBUS<b>:I2S:WLENgth"}, {"Level"=3, "Class Only"=FALSE, "Identifier"="RSRTX_ATTR_PROTOCOL_AUDIO_CHANNEL_ORDER", "Descriptive Name"="Protocol Audio Channel Order", "Data Type"=0, "Command"="BUS{SerialBus}:I2S:CHAN:ORD", "Access"=2, "Range Table"="rsrtx_rngAudioChannelOrder", "Read Callback"="", "Write Callback"="", "Supported Models"="RTM|RTA", "Instrument Options"="", "Flags"=0, "Help"="Defines if the left or the right channel is the first channel in the frame.\n\nAvailable Repeated Capabilities:\nSerialBus: SB1, SB2, SB3, SB4\r\n\nRemote-control command(s):\nBUS<b>:I2S:CHANnel:ORDer"}, {"Level"=3, "Class Only"=FALSE, "Identifier"="RSRTX_ATTR_PROTOCOL_AUDIO_BIT_ORDER", "Descriptive Name"="Protocol Audio Bit Order", "Data Type"=0, "Command"="BUS{SerialBus}:I2S:BORD", "Access"=2, "Range Table"="rsrtx_rngProtocolAudioBitOrder", "Read Callback"="", "Write Callback"="", "Supported Models"="RTM|RTA", "Instrument Options"="", "Flags"=0, "Help"="Select if the data of the messages starts with msb or lsb.\n\nAvailable Repeated Capabilities:\nSerialBus: SB1, SB2, SB3, SB4\r\n\nRemote-control command(s):\nBUS<b>:I2S:BORDer"}, {"Level"=3, "Class Only"=FALSE, "Identifier"="RSRTX_ATTR_PROTOCOL_AUDIO_CHANNEL_OFFSET", "Descriptive Name"="Protocol Audio Channel Offset", "Data Type"=0, "Command"="BUS{SerialBus}:I2S:CHAN:OFFS", "Access"=2, "Range Table"="rsrtx_rngAudioOffset", "Read Callback"="", "Write Callback"="", "Supported Models"="RTM|RTA", "Instrument Options"="", "Flags"=0, "Help"="Sets the number of bits between the channel start and the start of the audio word. The setting is available for left-justified data format and TDM audio signals.\n\nAvailable Repeated Capabilities:\nSerialBus: SB1, SB2, SB3, SB4\r\n\nRemote-control command(s):\nBUS<b>:I2S:CHANnel:OFFSet"}, {"Level"=3, "Class Only"=FALSE, "Identifier"="RSRTX_ATTR_PROTOCOL_AUDIO_CHANNEL_LENGTH", "Descriptive Name"="Protocol Audio Channel Length", "Data Type"=0, "Command"="BUS{SerialBus}:I2S:CHAN:LENG", "Access"=2, "Range Table"="", "Read Callback"="", "Write Callback"="", "Supported Models"="RTM|RTA", "Instrument Options"="", "Flags"=0, "Help"="Sets the number of bits in a channel block for right-justified data format and TDM audio signals.\n\nAvailable Repeated Capabilities:\nSerialBus: SB1, SB2, SB3, SB4\r\n\nRemote-control command(s):\nBUS<b>:I2S:CHANnel:LENGth"}, {"Level"=3, "Class Only"=FALSE, "Identifier"="RSRTX_ATTR_PROTOCOL_AUDIO_FRAME_OFFSET", "Descriptive Name"="Protocol Audio Frame Offset", "Data Type"=0, "Command"="BUS{SerialBus}:I2S:FOFF", "Access"=2, "Range Table"="rsrtx_rngAudioFrameOffset", "Read Callback"="", "Write Callback"="", "Supported Models"="RTM|RTA", "Instrument Options"="", "Flags"=0, "Help"="Sets the number of bits between the frame start and the start of the first channel of a TDM audio line. Each FSYNC edge restarts the offset count.\n\nAvailable Repeated Capabilities:\nSerialBus: SB1, SB2, SB3, SB4\r\n\nRemote-control command(s):\nBUS<b>:I2S:FOFFset"}, {"Level"=3, "Class Only"=FALSE, "Identifier"="RSRTX_ATTR_PROTOCOL_AUDIO_TDM_CHANNELS", "Descriptive Name"="Protocol Audio TDM Channels", "Data Type"=0, "Command"="BUS{SerialBus}:I2S:CHAN:TDMC", "Access"=2, "Range Table"="rsrtx_rngAudioTDMChannels", "Read Callback"="", "Write Callback"="", "Supported Models"="RTM|RTA", "Instrument Options"="", "Flags"=0, "Help"="Sets the number of channels transmitted on the TDM audio line.\n\nAvailable Repeated Capabilities:\nSerialBus: SB1, SB2, SB3, SB4\r\n\nRemote-control command(s):\nBUS<b>:I2S:CHANnel:TDMCount"}, {"Level"=3, "Class Only"=FALSE, "Identifier"="RSRTX_ATTR_PROTOCOL_AUDIO_SELECTED_FRAME", "Descriptive Name"="Protocol Audio Selected Frame", "Data Type"=0, "Command"="", "Access"=2, "Range Table"="", "Read Callback"="", "Write Callback"="", "Supported Models"="", "Instrument Options"="", "Flags"=0, "Help"="Sets selector repeated capability Frame.\n\nAvailable Repeated Capabilities:\nNone\n\nRemote-control command(s):\n"}, {"Level"=3, "Class Only"=FALSE, "Identifier"="RSRTX_ATTR_PROTOCOL_AUDIO_FRAME_COUNT", "Descriptive Name"="Protocol Audio Frame Count", "Data Type"=0, "Command"="BUS{SerialBus}:I2S:FCO?", "Access"=0, "Range Table"="", "Read Callback"="", "Write Callback"="", "Supported Models"="RTM|RTA", "Instrument Options"="", "Flags"=0, "Help"="Queries the number of decoded frames.\n\nAvailable Repeated Capabilities:\nSerialBus: SB1, SB2, SB3, SB4\r\n\nRemote-control command(s):\nBUS<b>:I2S:FCOunt?"}, {"Level"=3, "Class Only"=FALSE, "Identifier"="RSRTX_ATTR_PROTOCOL_AUDIO_FRAME_STATUS", "Descriptive Name"="Protocol Audio Frame Status", "Data Type"=0, "Command"="BUS{SerialBus}:I2S:FRAM<Frame>:STAT?", "Access"=0, "Range Table"="rsrtx_rngAudioFrameStatus", "Read Callback"="rsrtx_FormatAudioFrameRepCapInt_ReadCallback.vi", "Write Callback"="", "Supported Models"="RTM|RTA", "Instrument Options"="", "Flags"=0, "Help"="Returns the overall state of the frame.\n\nAvailable Repeated Capabilities:\nSerialBus: SB1, SB2, SB3, SB4\r\n\nRemote-control command(s):\nBUS<b>:I2S:FRAMe<n>:STATe?"}, {"Level"=3, "Class Only"=FALSE, "Identifier"="RSRTX_ATTR_PROTOCOL_AUDIO_FRAME_START", "Descriptive Name"="Protocol Audio Frame Start", "Data Type"=1, "Command"="BUS{SerialBus}:I2S:FRAM<Frame>:STAR?", "Access"=0, "Range Table"="", "Read Callback"="rsrtx_FormatAudioFrameRepCapReal_ReadCallback.vi", "Write Callback"="", "Supported 
